vi "Get_INI_Main_Section.vi"(0 "name or relative path":string="ModisEdge.ini", 1 "section":string="Main_Test", 2 "Sequence Path":path=path "C:/ModisEdge/Scope/Test Sequence/ModisEdge.ini", 3 "error in (no error)":errorcluster) -> (5 "Calibrator COM Port":string="COM12", 6 "DMM COM Port":string="COM2", 7 "AlwaysPrint":bool, 8 "error out":errorcluster)   [LabVIEW 2015]
uses:
  <vilib>/Utility/config.llb/Read Key (String).vi
  <vilib>/Utility/config.llb/Read Key (Boolean).vi
  <vilib>/Utility/config.llb/NI_LVConfig.lvlib
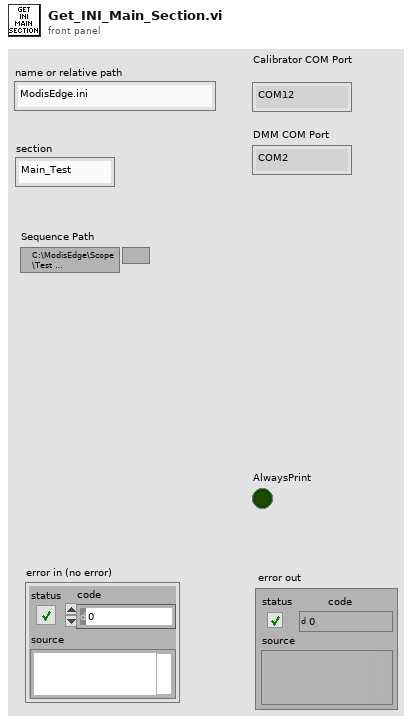
[diagram p1: front panel]
types:
  T1 = typedef "NI_LVConfig.lvlib/Config Data RefNum.ctl" = refnum<k1>
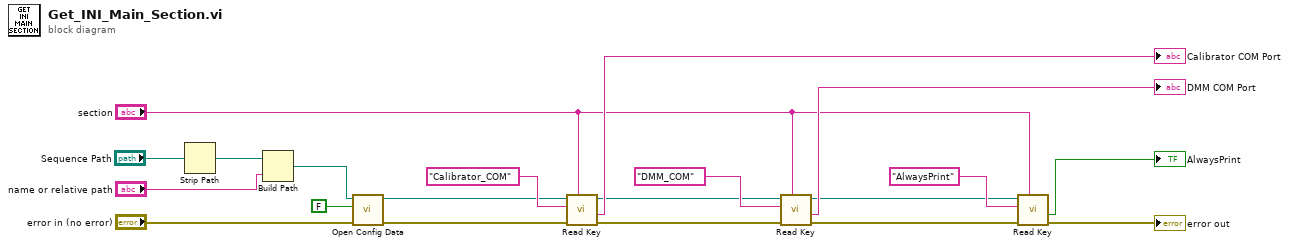
[diagram p0: block diagram]
diagram:
  n1 = Strip Path(path="Sequence Path") -> (stripped path=w1:path)  [unwired: 1 out]
  n2 = Build Path(base path=w1, name or relative path="name or relative path") -> (appended path=w7:path)
  n3 = call <vilib>:"Open Config Data.vi"("error in (no error)"="error in (no error)", "create file if necessary (T)"=FALSE, "configuration file path"=w7) -> ("error out"=w5:errorcluster, "refnum"=w4:T1)  [unwired: 6 in, 1 out]
  n4 = call-poly <vilib>:"Read Key.vi"("section"="section", "error in (no error)"=w5, "key"="Calibrator_COM", "refnum"=w4) -> ("error out"=w13:errorcluster, "value"=→"Calibrator COM Port":string, "refnum out"=w12:T1)  [unwired: 4 in, 1 out]
  n5 = call-poly <vilib>:"Read Key.vi"("section"="section", "error in (no error)"=w13, "key"="DMM_COM", "refnum"=w12) -> ("error out"=w11:errorcluster, "value"=→"DMM COM Port":string, "refnum out"=w10:T1)  [unwired: 4 in, 1 out]
  n6 = call-poly <vilib>:"Read Key.vi"("section"="section", "error in (no error)"=w11, "key"="AlwaysPrint", "refnum"=w10) -> ("error out"=→"error out":errorcluster, "value"=→"AlwaysPrint":bool)  [unwired: 4 in, 2 out]
